vi "RenameFilesSubVI.vi"(8 "Error In":errorcluster, 11 "FilePath":path) -> (0 "error out":errorcluster, 3 "new path":path)   [LabVIEW 2017]
uses:
  <vilib>/regexp/Match Regular Expression.xnode
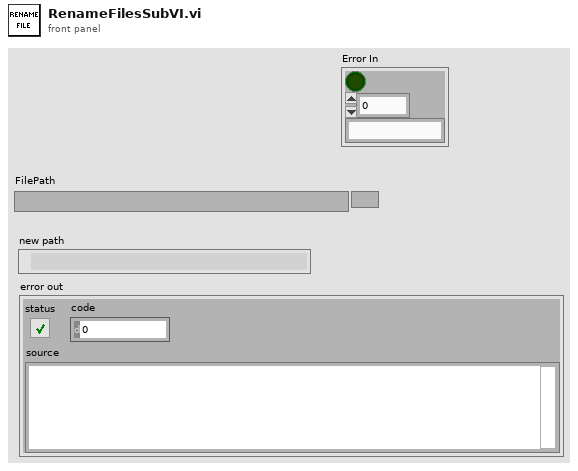
[diagram p1: front panel]
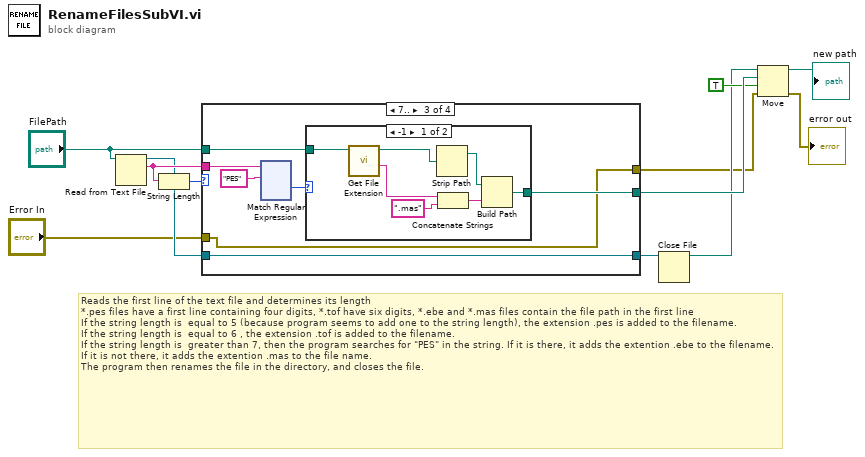
[diagram p0: block diagram]
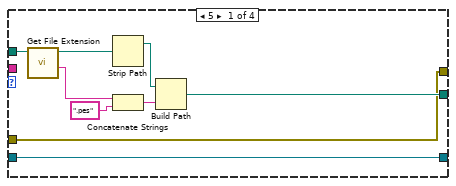
[diagram p2: hidden frame]
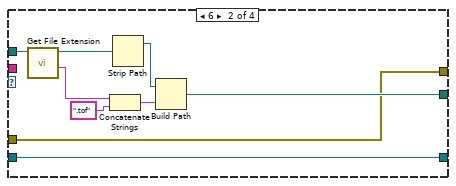
[diagram p3: hidden frame]
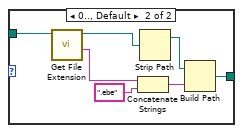
[diagram p4: hidden frame]
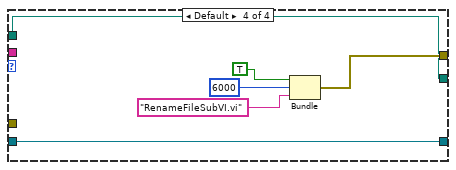
[diagram p5: hidden frame]
diagram:
  # "Reads the first line of the text file and determines its length\n*.pes files have a first line containing four digits, *.tof have six digits, *.ebe and *.mas files contain the file path in the first line\nIf the string length is  equal to 5 (because program seems to add one to the string length), the extension .pes is added to the filename.\nIf the string length is  equal to 6 , the extension .tof is added to the filename.\nIf the string length is  greater than 7, then the program searches for \"PES\" in the string. If it is there, it adds the extention .ebe to the filename. If it is not there, it adds the extention .mas to the file name.   \nThe program then renames the file in the directory, and closes the file."
  n1 = Read from Text File(file (use dialog)="FilePath") -> (refnum out=w8:refnum<file>, text=w10:string)  [unwired: 3 in, 2 out]
  n2 = String Length(string=w10) -> (length=w9:i32)
  n3 = case shown="7.." w9 {
    tunnel: [w15 w25 w33 w166] -> w11
    tunnel: "FilePath" -> [w16 w24 w34 w166]
    tunnel: w10 -> [_ _ w35 _]
    tunnel: w8 -> [w14 w23 w32 w167]
    tunnel: [w14 w23 w32 w167] -> w7
    tunnel: [w13 w22 w31 w168] -> w2
    tunnel: "Error In" -> [w13 w22 w31 _]
    frame 5 {
      n4 = call <vilib>:"Get File Extension.vi"("file"=w16) -> ("filename without extension"=w19:string, "dup file"=w18:path)  [unwired: 6 in, 3 out]
      n5 = Strip Path(path=w18) -> (stripped path=w17:path)  [unwired: 1 out]
      n6 = Concatenate Strings(w19, ".pes") -> (w20:string)
      n7 = Build Path(base path=w17, name or relative path=w20) -> (appended path=w15:path)
    }
    frame 6 {
      n8 = call <vilib>:"Get File Extension.vi"("file"=w24) -> ("filename without extension"=w28:string, "dup file"=w27:path)  [unwired: 6 in, 3 out]
      n9 = Concatenate Strings(w28, ".tof") -> (w29:string)
      n10 = Strip Path(path=w27) -> (stripped path=w26:path)  [unwired: 1 out]
      n11 = Build Path(base path=w26, name or relative path=w29) -> (appended path=w25:path)
    }
    frame 7.. {
      n12 = xnode "Match Regular Expression"("input string"=w35, "regular expression"="PES") -> ("offset past match"=w36:i32)  [unwired: 4 in, 4 out]
      n13 = case shown="-1" w36 {
        tunnel: w34 -> [w152 w164]
        tunnel: [w153 w165] -> w33
        frame -1 {
          n14 = call <vilib>:"Get File Extension.vi"("file"=w152) -> ("filename without extension"=w156:string, "dup file"=w155:path)  [unwired: 6 in, 3 out]
          n15 = Strip Path(path=w155) -> (stripped path=w154:path)  [unwired: 1 out]
          n16 = Concatenate Strings(w156, ".mas") -> (w157:string)
          n17 = Build Path(base path=w154, name or relative path=w157) -> (appended path=w153:path)
        }
        frame 0.., Default {
          n18 = call <vilib>:"Get File Extension.vi"("file"=w164) -> ("filename without extension"=w161:string, "dup file"=w160:path)  [unwired: 6 in, 3 out]
          n19 = Concatenate Strings(w161, ".ebe") -> (w162:string)
          n20 = Strip Path(path=w160) -> (stripped path=w159:path)  [unwired: 1 out]
          n21 = Build Path(base path=w159, name or relative path=w162) -> (appended path=w165:path)
        }
      }
    }
    frame Default {
      n22 = Bundle(TRUE, 6000, "RenameFileSubVI.vi") -> (w168:errorcluster)  [unwired: 1 in]
    }
  }
  n23 = Close File(refnum=w7) -> (path=w3:path)  [unwired: 1 in, 1 out]
  n24 = Move(source path=w3, error in=w2, 9:TRUE ("overwrite (F)"), 10:w11) -> (error out=→"error out":errorcluster, 3:→"new path":path)  [unwired: 1 in, 1 out]
